vi "DigitalOutCommand.vi"(2 "error in":errorcluster, 3 "Component ID":u16(ring) items=["left_itb_light_inner", "right_itb_light_inner", "torso_left_itb_light_inner", "torso_right_itb_light_inner", "left_itb_light_outer", "right_itb_light_outer", "torso_left_itb_light_outer", "torso_right_itb_light_outer", ""], 4 "State":bool, 5 "node":string) -> (0 "error out":errorcluster)   [LabVIEW 2012]
doc: "Write digital output to Baxters"
uses:
  <userlib>/ROSforLV/ROS/Code/Console/Servers/ServerSubs/TopicDef.ctl
  <userlib>/ROSforLV/ROS/Code/SubVIs/_ROSDirection.ctl
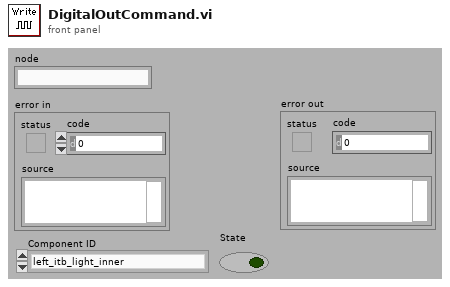
[diagram p1: front panel]
types:
  T1 = typedef "TopicDef.ctl" = cluster{"Topic":string, "Type":string, "Action":T2, "Update (ms)":u16, "queue size":u16}
  T2 = typedef "_ROSDirection.ctl" = enum16{"Node", "Publisher", "Subscriber", "Service Client"}
  T3 = typedef "_ROSControl.ctl" = cluster{"topic port":u16, "Node":string, "topic":string, "type":string, "node port":u16, "error ":errorcluster, "Direction":T2, "Update (ms)":u16, "queue size":u16}
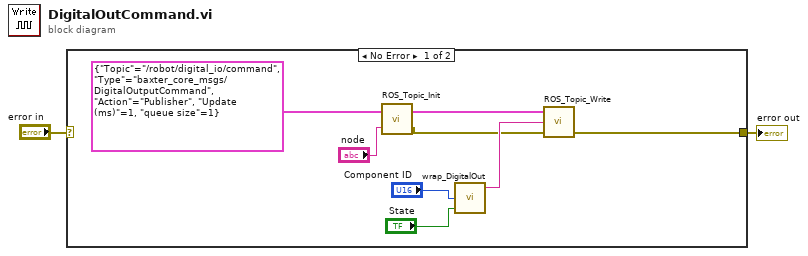
[diagram p0: block diagram]
diagram:
  n1 = case shown="No Error" "error in" {
    selector: "error in" -> [_ w11]
    tunnel: [w4 w11] -> w2
    frame No Error {
      n2 = call <userlib>:"ROS_Topic_Init.vi"("node"="node", "Definitions"=T1 {"Topic"="/robot/digital_io/command", "Type"="baxter_core_msgs/DigitalOutputCommand", "Action"=enum."Publisher", "Update (ms)"=1, "queue size"=1}) -> ("error out"=w3:errorcluster, "ROS out"=w10:T3)
      n3 = call <userlib>:"wrap_DigitalOut.vi"("State"="State", "Component ID"="Component ID") -> ("msg out"=w5:string)  [unwired: 3 in]
      n4 = call <userlib>:"ROS_Topic_Write.vi"("error in (no error)"=w3, "Msg in"=w5, "ROS in"=w10) -> ("error out"=w4:errorcluster)  [unwired: 1 in, 1 out]
    }
    frame Error {
    }
  }
  "error out" <- w2
